vi "Homing.vi"(0 "PWM2 in":dbl, 1 "PWM1 in":dbl, 2 "PosicionM1":dbl, 3 "PosicionM2":dbl, 4 "Contador":dbl, 5 "Enum":T1(ring), 6 "Home":bool, 7 "SensorM2":bool, 9 "SensorM1":bool) -> (20 "Estado":T1(ring), 21 "contador+1":dbl, 22 "PWM1":dbl, 23 "PWM2":dbl)   [LabVIEW 2018]
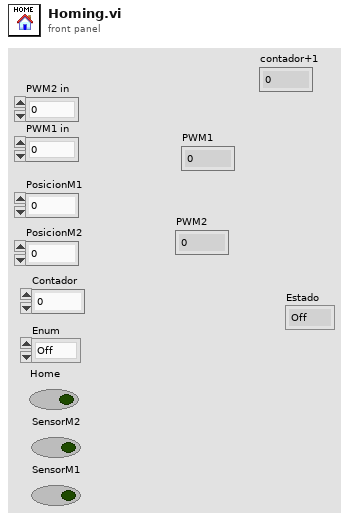
[diagram p1: front panel]
types:
  T1 = enum16{"Off", "Codo1", "ResetCodo1", "Codo2", "ResetCodo2", "Hombro1", "ResetHombro1", "Hombro2", "ResetHombro2"}
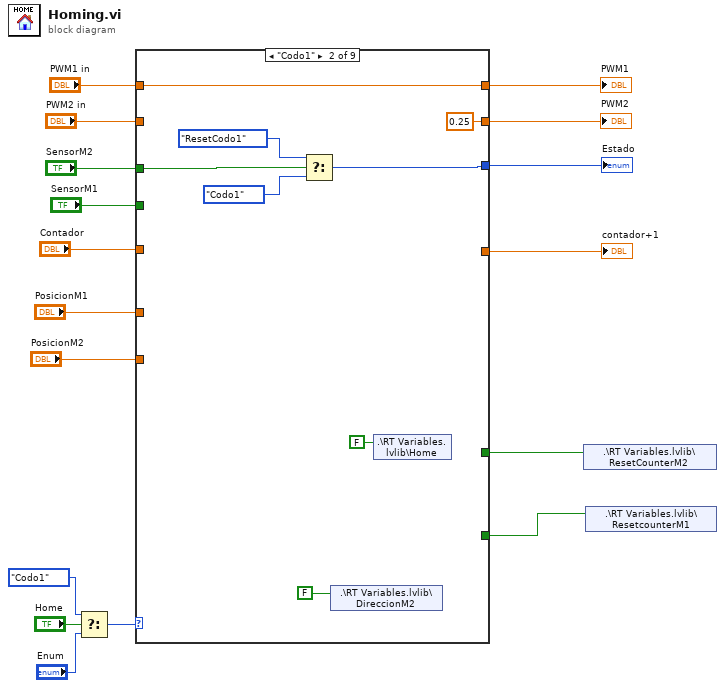
[diagram p0: block diagram]
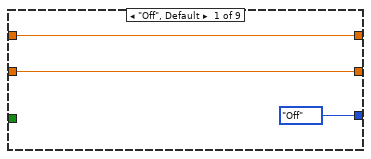
[diagram p2: hidden frame]
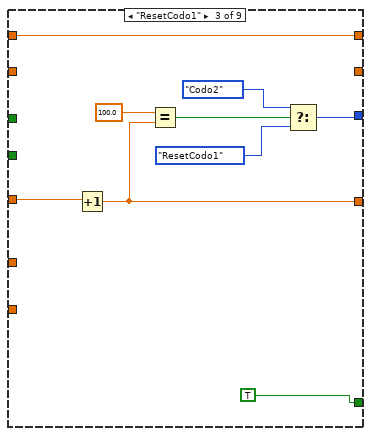
[diagram p3: hidden frame]
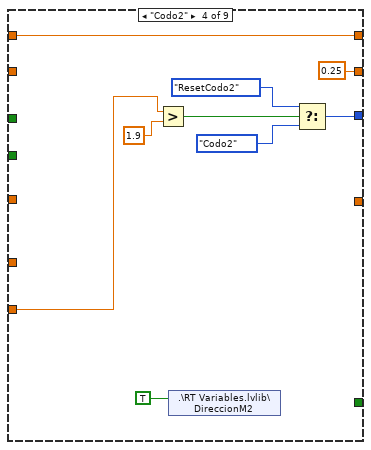
[diagram p4: hidden frame]
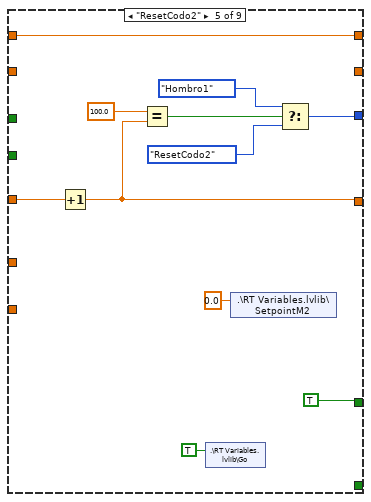
[diagram p5: hidden frame]
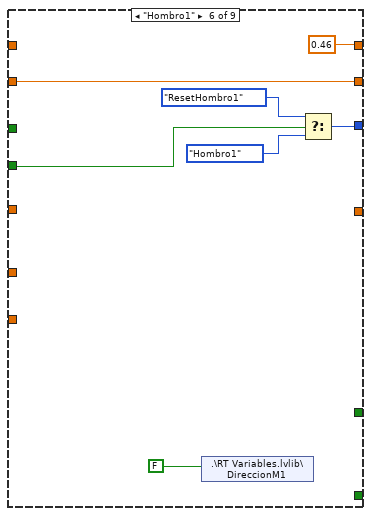
[diagram p6: hidden frame]
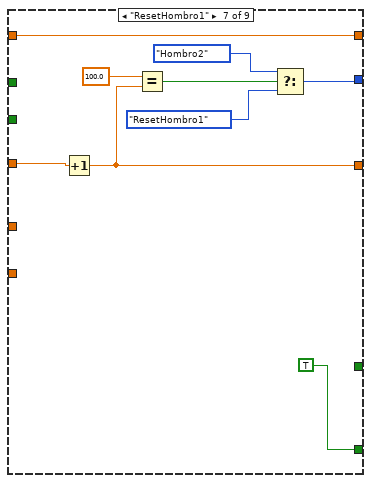
[diagram p7: hidden frame]
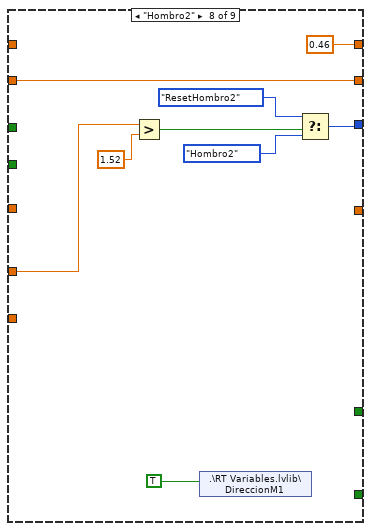
[diagram p8: hidden frame]
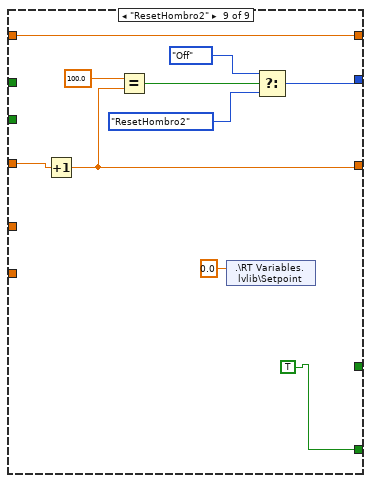
[diagram p9: hidden frame]
diagram:
  n1 = Select(t=T1."Codo1" ("Enum"), s="Home", f="Enum") -> (s? t:f=w16:T1)
  n2 = case shown="\"Codo1\"" w16 {
    tunnel: [T1."Off" ("Enum") w24 w33 w44 w52 w62 w67 w80 w86] -> w14
    tunnel: [w19 w23 w29 w41 w48 0.46 ("PWM1 in") _ 0.46 ("PWM1 in") _] -> w13
    tunnel: [w18 0.25 ("PWM2 in") _ 0.25 ("PWM2 in") _ w59 w66 w77 w84] -> w12
    tunnel: "PWM1 in" -> [w19 w23 w29 w41 w48 _ _ _ _]
    tunnel: "PWM2 in" -> [w18 _ _ _ _ w59 w66 w77 w84]
    tunnel: "SensorM2" -> [_ w27 _ _ _ _ _ _ _]
    tunnel: [_ _ TRUE ("Boolean") _ TRUE ("Boolean") _ _ _ _] -> w7
    tunnel: "Contador" -> [_ _ w36 _ w51 _ w69 _ w88]
    tunnel: [_ _ w35 _ w50 _ w68 _ w87] -> w5
    tunnel: "SensorM1" -> [_ _ _ _ _ w60 _ _ _]
    tunnel: "PosicionM2" -> [_ _ _ w38 _ _ _ _ _]
    tunnel: "PosicionM1" -> [_ _ _ _ _ _ _ w74 _]
    tunnel: [_ _ _ _ _ _ TRUE ("Boolean") _ TRUE ("Boolean")] -> w1
    frame "Off", Default {
    }
    frame "Codo1" {
      n3 = Select(t=T1."ResetCodo1" ("Enum"), s=w27, f=T1."Codo1" ("Enum")) -> (s? t:f=w24:T1)
      n4 = shared-variable ".\\RT Variables.lvlib\\DireccionM2"(FALSE ("Boolean")) -> ()  [unwired: 1 in, 1 out]
      n5 = shared-variable ".\\RT Variables.lvlib\\Home"(FALSE ("Home")) -> ()  [unwired: 1 in, 1 out]
    }
    frame "ResetCodo1" {
      n6 = Increment(x=w36) -> (x+1=w35:dbl)
      n7 = Equal?(x=100.0, y=w35) -> (x = y?=w30:bool)
      n8 = Select(t=T1."Codo2" ("Enum"), s=w30, f=T1."ResetCodo1" ("Enum")) -> (s? t:f=w33:T1)
    }
    frame "Codo2" {
      n9 = Greater?(x=w38, y=1.9 ("x")) -> (0:w42:bool)
      n10 = shared-variable ".\\RT Variables.lvlib\\DireccionM2"(TRUE ("Boolean")) -> ()  [unwired: 1 in, 1 out]
      n11 = Select(t=T1."ResetCodo2" ("Enum"), s=w42, f=T1."Codo2" ("Enum")) -> (s? t:f=w44:T1)
    }
    frame "ResetCodo2" {
      n12 = Increment(x=w51) -> (x+1=w50:dbl)
      n13 = Equal?(x=100.0, y=w50) -> (x = y?=w54:bool)
      n14 = shared-variable ".\\RT Variables.lvlib\\Go"(TRUE ("Go")) -> ()  [unwired: 1 in, 1 out]
      n15 = shared-variable ".\\RT Variables.lvlib\\SetpointM2"(0.0 ("SetpointM2")) -> ()  [unwired: 1 in, 1 out]
      n16 = Select(t=T1."Hombro1" ("Enum"), s=w54, f=T1."ResetCodo2" ("Enum")) -> (s? t:f=w52:T1)
    }
    frame "Hombro1" {
      n17 = shared-variable ".\\RT Variables.lvlib\\DireccionM1"(FALSE ("Boolean")) -> ()  [unwired: 1 in, 1 out]
      n18 = Select(t=T1."ResetHombro1" ("Enum"), s=w60, f=T1."Hombro1" ("Enum")) -> (s? t:f=w62:T1)
    }
    frame "ResetHombro1" {
      n19 = Increment(x=w69) -> (x+1=w68:dbl)
      n20 = Equal?(x=100.0, y=w68) -> (x = y?=w70:bool)
      n21 = Select(t=T1."Hombro2" ("Enum"), s=w70, f=T1."ResetHombro1" ("Enum")) -> (s? t:f=w67:T1)
    }
    frame "Hombro2" {
      n22 = Greater?(x=w74, y=1.52 ("x")) -> (0:w78:bool)
      n23 = shared-variable ".\\RT Variables.lvlib\\DireccionM1"(TRUE ("Boolean")) -> ()  [unwired: 1 in, 1 out]
      n24 = Select(t=T1."ResetHombro2" ("Enum"), s=w78, f=T1."Hombro2" ("Enum")) -> (s? t:f=w80:T1)
    }
    frame "ResetHombro2" {
      n25 = Increment(x=w88) -> (x+1=w87:dbl)
      n26 = Equal?(x=100.0, y=w87) -> (x = y?=w89:bool)
      n27 = shared-variable ".\\RT Variables.lvlib\\Setpoint"(0.0 ("SetpointM1")) -> ()  [unwired: 1 in, 1 out]
      n28 = Select(t=T1."Off" ("Enum"), s=w89, f=T1."ResetHombro2" ("Enum")) -> (s? t:f=w86:T1)
    }
  }
  "Estado" <- w14
  "PWM1" <- w13
  "PWM2" <- w12
  "contador+1" <- w5
  n29 = shared-variable ".\\RT Variables.lvlib\\ResetCounterM2"(w7) -> ()  [unwired: 1 in, 1 out]
  n30 = shared-variable ".\\RT Variables.lvlib\\ResetcounterM1"(w1) -> ()  [unwired: 1 in, 1 out]
